vi "Continuous Acquisition Sample.vi"(8 "Error In":errorcluster, 9 "Sample Rate (HZ)":u16, 10 "Samples to Read":u16, 11 "ChipKit Resource":T1={"COM Port"="", "Board Type"=enum."ChipKit uC32", "Connection Type"=enum."USB / Serial", "Baud Rate (115200)"=0, "Bytes Per Packet (15)"=15, "DI Port Num Pins"=0, "DO Port Num Pins"=0}) -> (0 "Error Out":errorcluster, 2 "Data":dbl[](array[numeric]), 3 "ChipKit Resource":T1={"COM Port"="", "Board Type"=enum."ChipKit uC32", "Connection Type"=enum."USB / Serial", "Baud Rate (115200)"=0, "Bytes Per Packet (15)"=15, "DI Port Num Pins"=0, "DO Port Num Pins"=0})   [LabVIEW 2011, in "LabVIEW Interface for ChipKit.lvlib"]
doc: "Returns the number of samples specified at the rate specified. At high sample rates this VI must executed frequently enough to keep up with the samples available at the serial port."
uses:
  LabVIEW Interface for ChipKit.lvlib
  Private/Type Defs/Chipkit Resource.ctl
  Private/Type Defs/Board Type.ctl
  Private/Type Defs/Connection Type.ctl
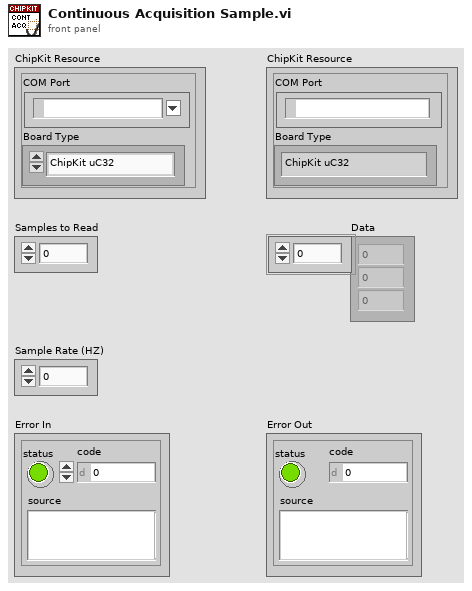
[diagram p1: front panel]
types:
  T1 = typedef "LabVIEW Interface for ChipKit.lvlib/Chipkit Resource.ctl" = cluster{"COM Port":refnum<visa-resource-name>, "Board Type":T2, "Connection Type":T3, "Baud Rate (115200)":u32, "Bytes Per Packet (15)":u32, "DI Port Num Pins":i32, "DO Port Num Pins":i32}
  T2 = typedef "LabVIEW Interface for ChipKit.lvlib/Board Type.ctl" = enum16{"ChipKit uC32", "ChipKit Uno32", "ChipKit Max32"}
  T3 = typedef "LabVIEW Interface for ChipKit.lvlib/Connection Type.ctl" = enum8{"USB / Serial", "XBEE", "BlueSmirf (Bluetooth)"}
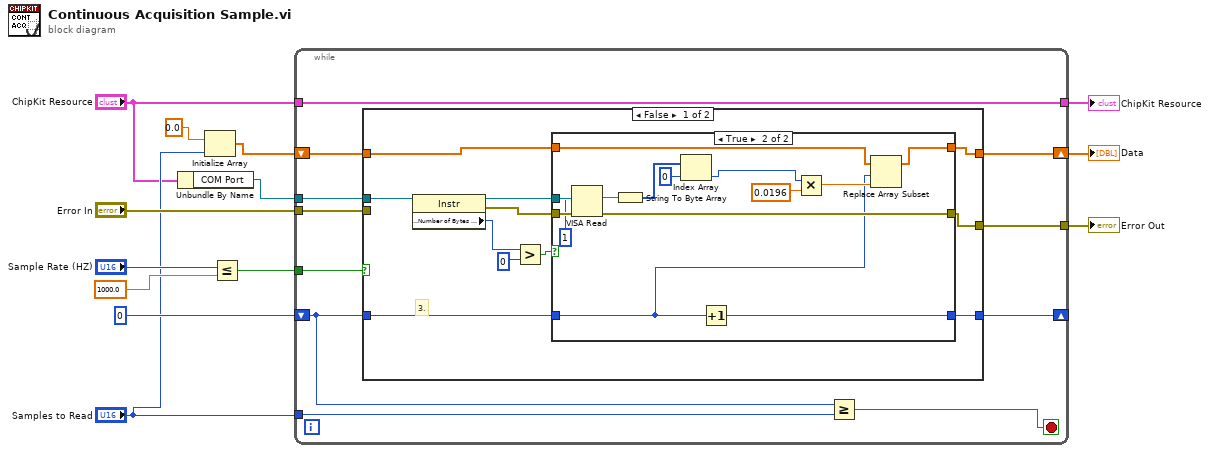
[diagram p0: block diagram]
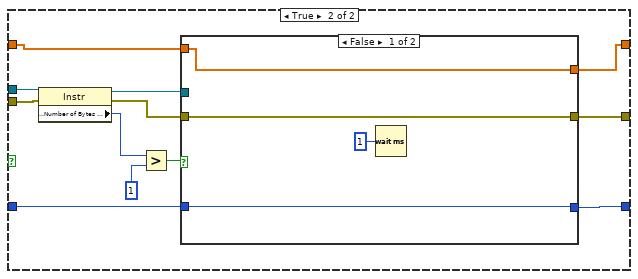
[diagram p3: hidden frame]
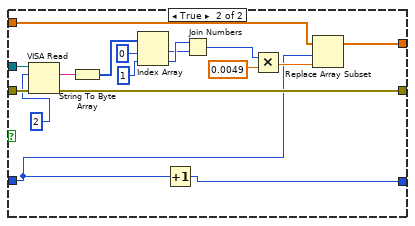
[diagram p4: hidden frame]
diagram:
  n1 = Unbundle By Name("ChipKit Resource") -> ("COM Port"=w8:refnum<visa-resource-name>)
  n2 = Initialize Array(0.0 ("element"), "Samples to Read") -> (w4:dbl[])
  n3 = Less Or Equal?(x="Sample Rate (HZ)", y=1000.0) -> (x <= y?=w10:bool)
  n4 = while {
    tunnel: "Error In" -> [w24]
    tunnel: w10 -> [w23]
    tunnel: [w22] -> w9
    tunnel: w8 -> [w21]
    shift-right: [w17] -> _
    shift-left: 0 -> [w18]
    tunnel: "Samples to Read" -> [w20]
    shift-right: [w15] -> w3
    shift-left: w4 -> [w16]
    tunnel: [w14] -> w1
    tunnel: "ChipKit Resource" -> [w14]
    stop <- w19 stop-if-true
    # "3."
    n5 = case shown="False" w23 {
      tunnel: [w31 w63] -> w22
      tunnel: w21 -> [w30 w59]
      tunnel: w24 -> [_ w57]
      tunnel: w18 -> [w28 w56]
      tunnel: [w27 w55] -> w17
      tunnel: w16 -> [w26 w54]
      tunnel: [w25 w53] -> w15
      frame False {
        n6 = property class="Instr"(reference=w30) -> (reference out=w29:refnum<visa-resource-name>, error out=w32:errorcluster, "Serial Settings:Number of Bytes at Serial Port"=w33:u32)  [unwired: 1 in]
        n7 = Greater?(x=w33, y=u32 0) -> (0:w35:bool)
        n8 = case shown="True" w35 {
          tunnel: w32 -> [w38 w52]
          tunnel: [w38 w51] -> w31
          tunnel: w29 -> [_ w45]
          tunnel: w28 -> [w36 w41]
          tunnel: [w36 w43] -> w27
          tunnel: w26 -> [w37 w40]
          tunnel: [w37 w39] -> w25
          frame False {
          }
          frame True {
            n9 = VISA Read(VISA resource name=w45, byte count=1, error in (no error)=w52) -> (read buffer=w50:string, error out=w51:errorcluster)  [unwired: 2 out]
            n10 = String To Byte Array(string=w50) -> (unsigned byte array=w49:u8[])
            n11 = Index Array(array=w49, index=0) -> (element=w46:u8)
            n12 = Increment(x=w41) -> (x+1=w43:i32)
            n13 = Multiply(x=w46, y=0.0196) -> (x*y=w42:dbl)
            n14 = Replace Array Subset(array=w40, new element=w42, index=w41) -> (w39:dbl[])
          }
        }
      }
      frame True {
        n15 = property class="Instr"(reference=w59, error in=w57) -> (reference out=w58:refnum<visa-resource-name>, error out=w64:errorcluster, "Serial Settings:Number of Bytes at Serial Port"=w62:u32)
        n16 = Greater?(x=w62, y=u32 1) -> (0:w60:bool)
        n17 = case shown="False" w60 {
          tunnel: w64 -> [w68 w85]
          tunnel: [w68 w84] -> w63
          tunnel: w58 -> [_ w74]
          tunnel: w56 -> [w67 w72]
          tunnel: [w67 w71] -> w55
          tunnel: w54 -> [w66 w70]
          tunnel: [w66 w69] -> w53
          frame False {
            n18 = Wait (ms)(milliseconds to wait=u32 1) -> ()  [unwired: 1 out]
          }
          frame True {
            n19 = VISA Read(VISA resource name=w74, byte count=2, error in (no error)=w85) -> (read buffer=w83:string, error out=w84:errorcluster)  [unwired: 2 out]
            n20 = String To Byte Array(string=w83) -> (unsigned byte array=w82:u8[])
            n21 = Index Array(array=w82, index #1=0 ("index"), index #2=1 ("index")) -> (element #1=w77:u8, element #2=w78:u8)
            n22 = Increment(x=w72) -> (x+1=w71:i32)
            n23 = Join Numbers(hi=w78, lo=w77) -> ((hi.lo)=w76:u16)
            n24 = Multiply(x=w76, y=0.0049) -> (x*y=w73:dbl)
            n25 = Replace Array Subset(array=w70, new element=w73, index=w72) -> (w69:dbl[])
          }
        }
      }
    }
    n26 = Greater Or Equal?(x=w18, y=w20) -> (x >= y?=w19:bool)
  }
  "Error Out" <- w9
  "Data" <- w3
  "ChipKit Resource" <- w1
